vi "forceOutputState.vi"(8 "error in (no error)":errorcluster, 9 "data":T1(array[cluster]), 10 "physicalChannels":string[](array[string]), 11 "CQT_DDS in":refnum<class "CQT_DDS.lvclass">) -> (0 "error out":errorcluster, 3 "CQT_DDS out":refnum<class "CQT_DDS.lvclass">)   [LabVIEW 2011, in "CQT_DDS.lvclass"]
uses:
  CQT_DDS.lvclass
  CQT_DDS.lvclass/CQT_DDS.ctl
  C:/Program Files/National Instruments/LabVIEW 2011/instr.lib/CQT_DDS/DDSLibrary/20111109/CQTAD9958.dll
  Program Files/National Instruments/LabVIEW 2011/instr.lib/CQT_DDS/DDSLibrary/20111109/CQTAD9958.dll
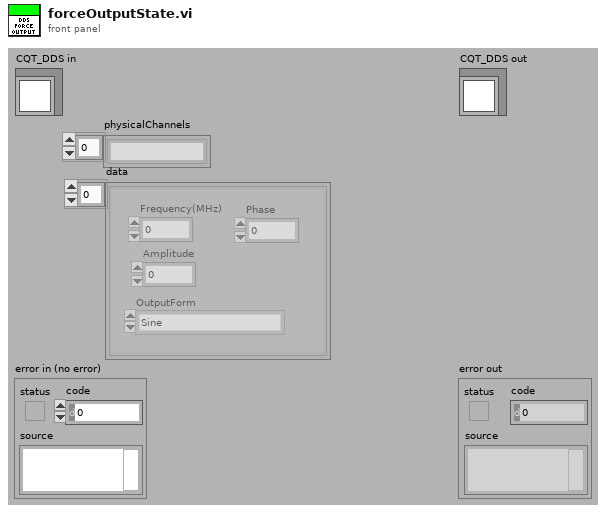
[diagram p1: front panel]
types:
  T1 = cluster{"Frequency(MHz)":dbl, "Amplitude":dbl, "Phase":dbl, "OutputForm":enum16{"Sine", "Square", "Triangle", "Arbitrary"}}[]
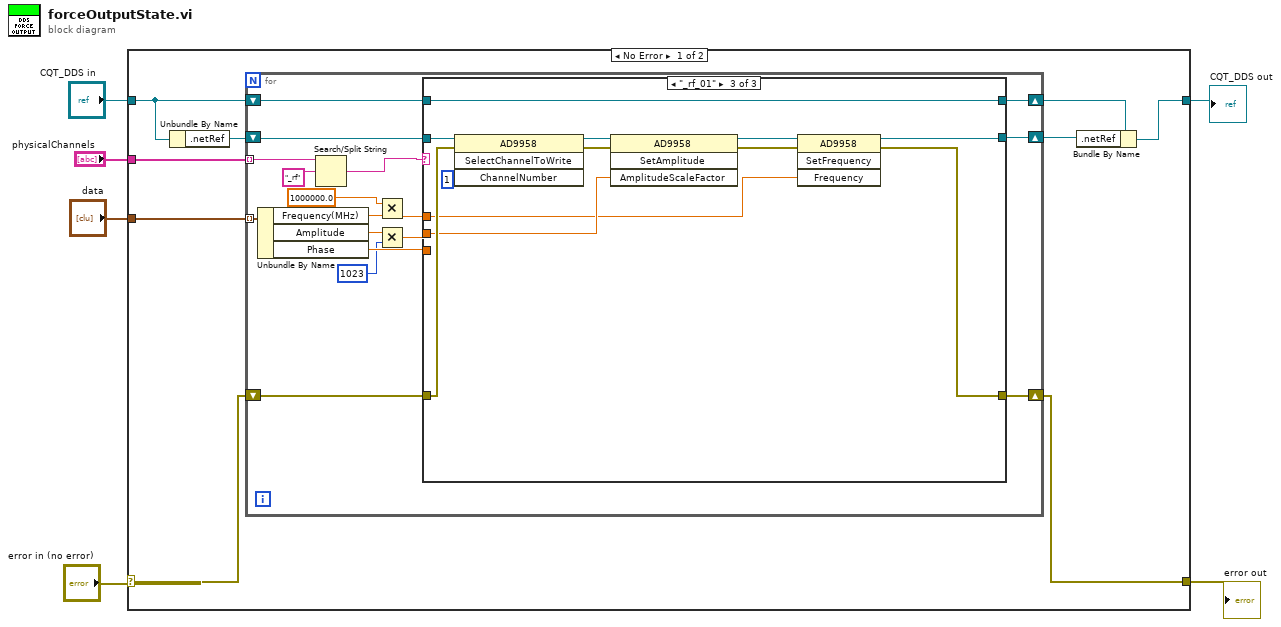
[diagram p0: block diagram]
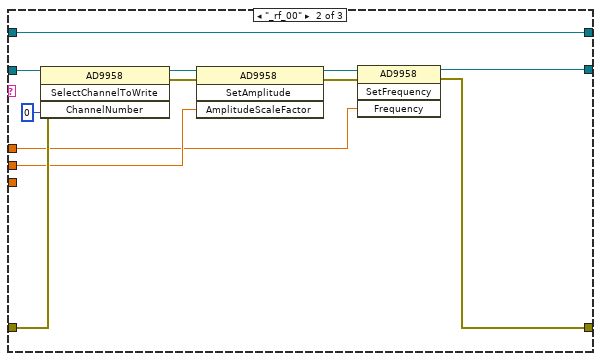
[diagram p3: hidden frame]
diagram:
  n1 = case shown="No Error" "error in (no error)" {
    selector: "error in (no error)" -> [w13 w60]
    tunnel: [w7 w61] -> w4
    tunnel: "CQT_DDS in" -> [w11 w61]
    tunnel: "physicalChannels" -> [w15 _]
    tunnel: "data" -> [w14 _]
    tunnel: [w12 w60] -> w1
    frame No Error {
      n2 = Unbundle By Name(w11) -> (".netRef"=w10:refnum<k24>)
      n3 = for {
        tunnel: w15 -> [w23] mode=indexing
        tunnel: w14 -> [w30] mode=indexing
        shift-right: [w32] -> w8
        shift-left: w11 -> [w31]
        shift-right: [w27] -> w12
        shift-left: w13 -> [w28]
        shift-right: [w25] -> w9
        shift-left: w10 -> [w26]
        n4 = Unbundle By Name(w30) -> ("Frequency(MHz)"=w20:dbl, "Amplitude"=w29:dbl, "Phase"=w24:dbl)
        n5 = Search/Split String(string=w23, search string/char (-)="_rf") -> (match + rest of string=w21:string)  [unwired: 1 in, 2 out]
        n6 = Multiply(x=1000000.0, y=w20) -> (x*y=w19:dbl)
        n7 = Multiply(x=w29, y=1023) -> (x*y=w17:dbl)
        n8 = case shown="\"_rf_01\"" w21 {
          tunnel: [w35 w47 w59] -> w32
          tunnel: w31 -> [w35 w47 w59]
          tunnel: w19 -> [_ w38 w49]
          tunnel: w17 -> [_ w41 w54]
          tunnel: w28 -> [w33 w44 w57]
          tunnel: [w33 w36 w50] -> w27
          tunnel: w26 -> [w34 w46 w58]
          tunnel: [w34 w37 w53] -> w25
          tunnel: w24 -> [_ _ _]
          frame Default {
            # "no such channel"
          }
          frame "_rf_00" {
            n9 = invoke class="AD9958" method="SelectChannelToWrite"(reference=w46, error in=w44, "ChannelNumber"=0) -> (reference out=w42:refnum<k24>, error out=w43:errorcluster)  [unwired: 1 in, 2 out]
            n10 = invoke class="AD9958" method="SetAmplitude"(reference=w42, error in=w43, "AmplitudeScaleFactor"=w41) -> (reference out=w40:refnum<k24>, error out=w39:errorcluster)  [unwired: 1 in, 2 out]
            n11 = invoke class="AD9958" method="SetFrequency"(reference=w40, error in=w39, "Frequency"=w38) -> (reference out=w37:refnum<k24>, error out=w36:errorcluster)  [unwired: 1 in, 2 out]
          }
          frame "_rf_01" {
            n12 = invoke class="AD9958" method="SelectChannelToWrite"(reference=w58, error in=w57, "ChannelNumber"=1) -> (reference out=w55:refnum<k24>, error out=w56:errorcluster)  [unwired: 1 in, 2 out]
            n13 = invoke class="AD9958" method="SetAmplitude"(reference=w55, error in=w56, "AmplitudeScaleFactor"=w54) -> (reference out=w52:refnum<k24>, error out=w51:errorcluster)  [unwired: 1 in, 2 out]
            n14 = invoke class="AD9958" method="SetFrequency"(reference=w52, error in=w51, "Frequency"=w49) -> (reference out=w53:refnum<k24>, error out=w50:errorcluster)  [unwired: 1 in, 2 out]
          }
        }
      }
      n15 = Bundle By Name(cluster=w8, ".netRef"=w9) -> (w7:refnum<class "CQT_DDS.lvclass">)
    }
    frame Error {
    }
  }
  "error out" <- w1
  "CQT_DDS out" <- w4
